vi "hardware_optpump.vi"(8 "error in":errorcluster, 10 "Pump?":bool) -> (0 "error out":errorcluster)   [LabVIEW 2012]
uses:
  <vilib>/DAQmx/write.llb/DAQmx Write (Digital Wfm 1Chan NSamp).vi
  <vilib>/Waveform/DWDTOps.llb/Digital Pattern Generator (Single Value).vi
  <vilib>/Waveform/DWDTOps.llb/DWDT Append Digital Samples.vi
  <vilib>/Waveform/DWDTOps.llb/DWDT Digital Size.vi
  <vilib>/DAQmx/create/channels.llb/DAQmx Create Channel (DO-Digital Output).vi
  <vilib>/DAQmx/configure/timing.llb/DAQmx Timing (Sample Clock).vi
  <vilib>/Waveform/DWDTOps.llb/DWDT Uncompress Digital.vi
  <vilib>/DAQmx/miscellaneous.llb/DAQmx Fill In Error Info.vi
  <resource>/objmgr/daqmx.rc
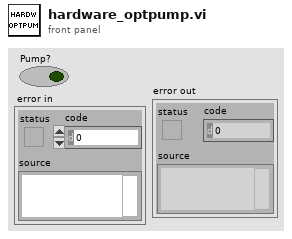
[diagram p1: front panel]
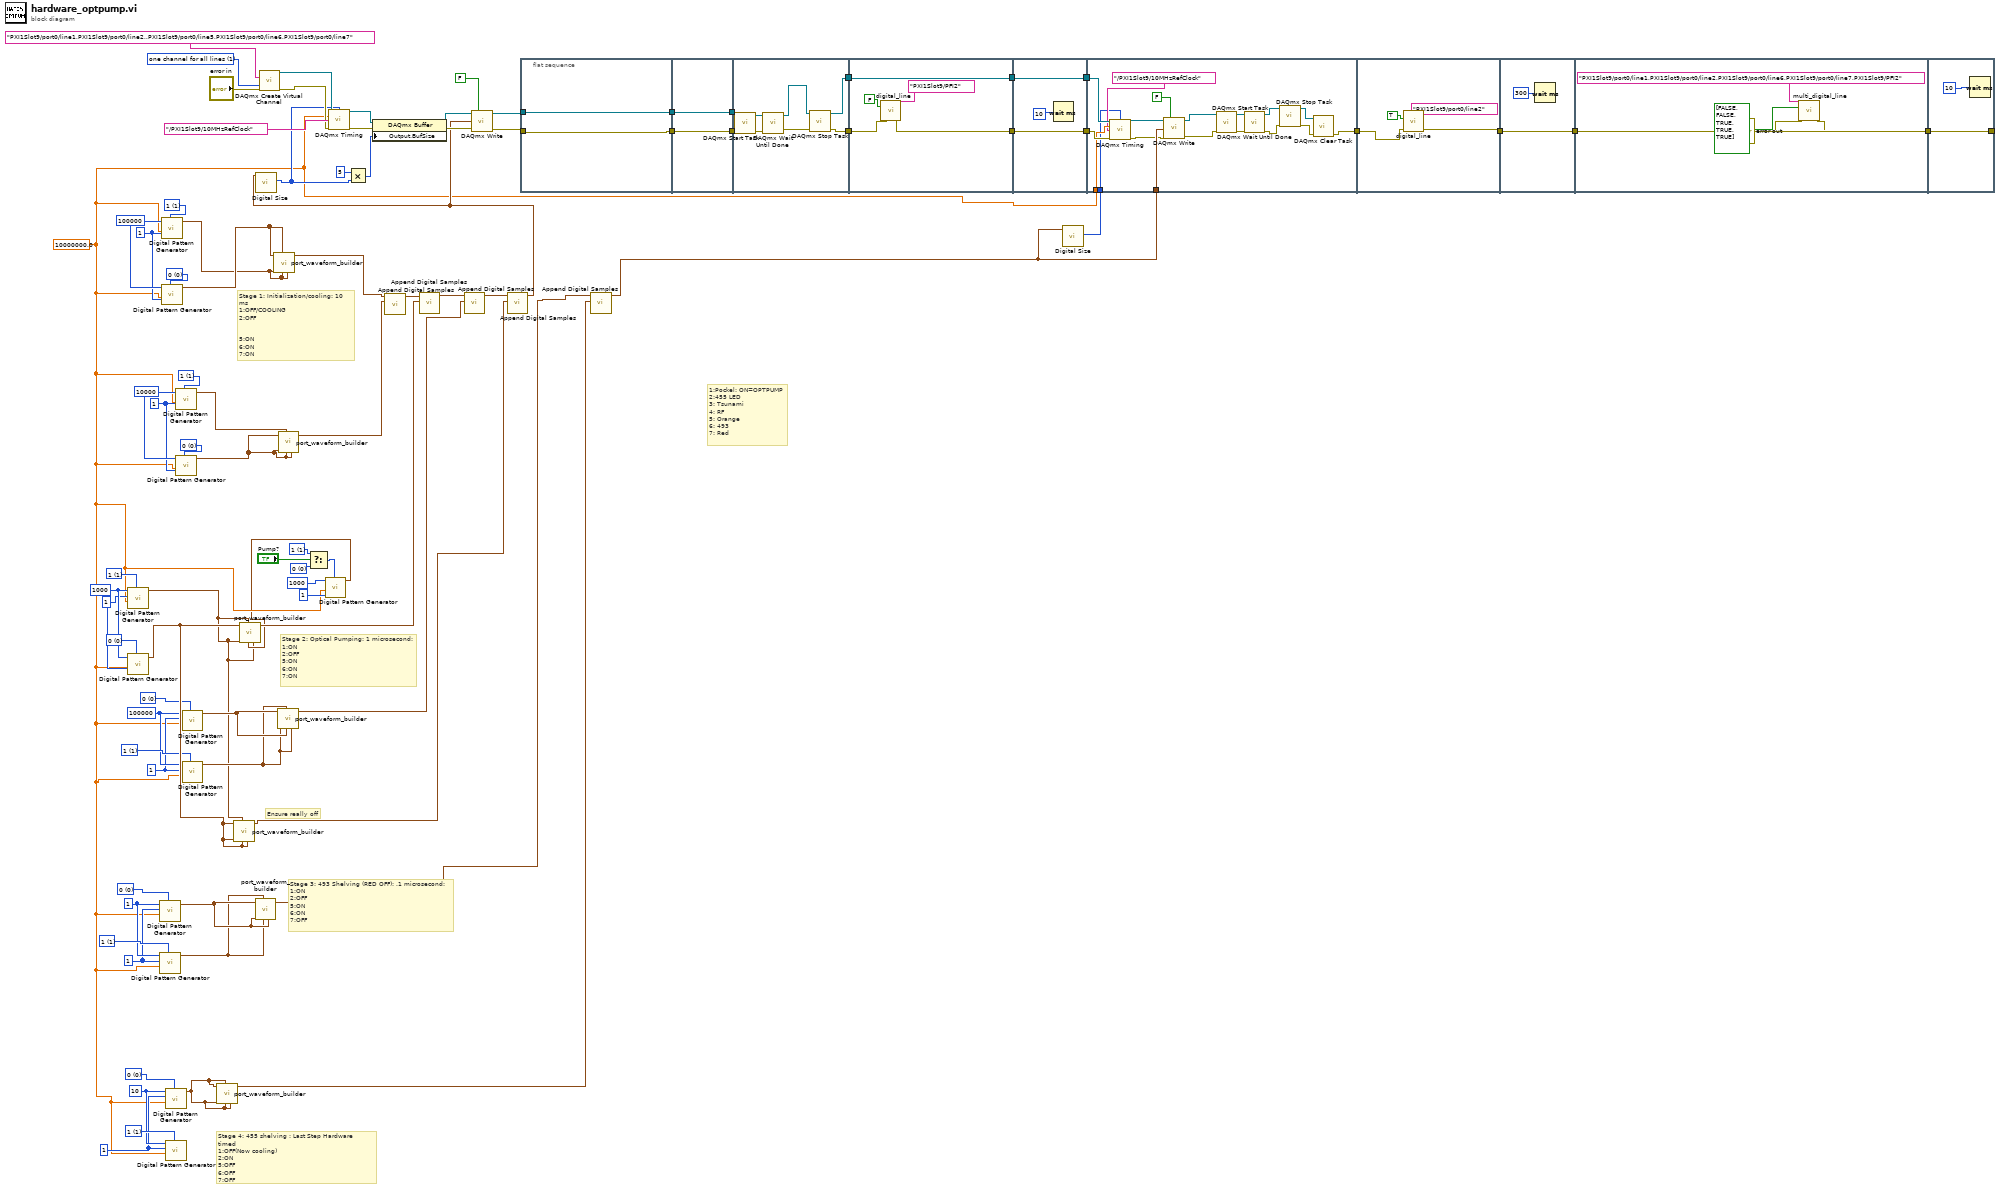
[diagram p0: block diagram]
diagram:
  w30 = u8 0 items=["0", "1", "Z", "L", "H", "X", "T", "V"] ("value")
  w28 = u32 1 ("number of signals")
  w29 = u32 100000 ("number of samples")
  w31 = u8 1 items=["0", "1", "Z", "L", "H", "X", "T", "V"] ("value")
  w44 = u8 0 items=["0", "1", "Z", "L", "H", "X", "T", "V"] ("value")
  w42 = u32 1 ("number of signals")
  w43 = u32 10000 ("number of samples")
  w45 = u8 1 items=["0", "1", "Z", "L", "H", "X", "T", "V"] ("value")
  w51 = u8 1 items=["0", "1", "Z", "L", "H", "X", "T", "V"] ("value")
  w50 = u8 0 items=["0", "1", "Z", "L", "H", "X", "T", "V"] ("value")
  w62 = u8 0 items=["0", "1", "Z", "L", "H", "X", "T", "V"] ("value")
  w60 = u32 1 ("number of signals")
  w61 = u32 10 ("number of samples")
  w63 = u8 1 items=["0", "1", "Z", "L", "H", "X", "T", "V"] ("value")
  w66 = u8 0 items=["0", "1", "Z", "L", "H", "X", "T", "V"] ("value")
  w64 = u32 1 ("number of signals")
  w65 = u32 1 ("number of samples")
  w67 = u8 1 items=["0", "1", "Z", "L", "H", "X", "T", "V"] ("value")
  w72 = u8 0 items=["0", "1", "Z", "L", "H", "X", "T", "V"] ("value")
  w68 = u32 1 ("number of signals")
  w69 = u32 1000 ("number of samples")
  w73 = u8 1 items=["0", "1", "Z", "L", "H", "X", "T", "V"] ("value")
  w74 = u8 0 items=["0", "1", "Z", "L", "H", "X", "T", "V"] ("value")
  w70 = u32 1 ("number of signals")
  w71 = u32 100000 ("number of samples")
  w75 = u8 1 items=["0", "1", "Z", "L", "H", "X", "T", "V"] ("value")
  w80 = 1 items=["one channel for each line", "one channel for all lines"] ("line grouping")
  w7 = 10000000.0 ("rate")
  # "Ensure really off"
  # "Stage 4: 455 shelving : Last Step Hardware timed\n1:OFF(Now cooling)\n2:ON\n5:OFF\n6:OFF\n7:OFF"
  # "Stage 3: 493 Shelving (RED OFF): .1 microsecond: \n1:ON\n2:OFF\n5:ON\n6:ON\n7:OFF"
  # "Stage 2: Optical Pumping: 1 microsecond: \n1:ON\n2:OFF\n5:ON\n6:ON\n7:ON"
  # "Stage 1: Initialization/cooling: 10 ms\n1:OFF/COOLING\n2:OFF\n\n\n5:ON\n6:ON\n7:ON"
  # "1:Pockel: ON=OPTPUMP\n2:455 LED\n3: Tsunami\n4: RF\n5: Orange\n6: 493\n7: Red"
  n1 = call-poly <vilib>:"Digital Pattern Generator.vi"("value"=w73, "sample rate"=w7, "number of signals"=w68, "number of samples"=w69) -> ("digital waveform"=w2:digitalwaveform)  [unwired: 6 in, 1 out]
  n2 = call-poly <vilib>:"Digital Pattern Generator.vi"("value"=w72, "sample rate"=w7, "number of signals"=w68, "number of samples"=w69) -> ("digital waveform"=w36:digitalwaveform)  [unwired: 6 in, 1 out]
  n3 = call-poly <vilib>:"Digital Pattern Generator.vi"("value"=w66, "sample rate"=w7, "number of signals"=w64, "number of samples"=w65) -> ("digital waveform"=w4:digitalwaveform)  [unwired: 6 in, 1 out]
  n4 = call-poly <vilib>:"Digital Pattern Generator.vi"("value"=w67, "sample rate"=w7, "number of signals"=w64, "number of samples"=w65) -> ("digital waveform"=w1:digitalwaveform)  [unwired: 6 in, 1 out]
  n5 = call-poly <vilib>:"Digital Pattern Generator.vi"("value"=w75, "sample rate"=w7, "number of signals"=w70, "number of samples"=w71) -> ("digital waveform"=w53:digitalwaveform)  [unwired: 6 in, 1 out]
  n6 = call-poly <vilib>:"Digital Pattern Generator.vi"("value"=w74, "sample rate"=w7, "number of signals"=w70, "number of samples"=w71) -> ("digital waveform"=w54:digitalwaveform)  [unwired: 6 in, 1 out]
  n7 = call-poly <vilib>:"Digital Pattern Generator.vi"("value"=w62, "sample rate"=w7, "number of signals"=w60, "number of samples"=w61) -> ("digital waveform"=w32:digitalwaveform)  [unwired: 6 in, 1 out]
  n8 = call-poly <vilib>:"Digital Pattern Generator.vi"("value"=w63, "sample rate"=w7, "number of signals"=w60, "number of samples"=w61) -> ()  [unwired: 6 in, 2 out]
  n9 = call-poly <vilib>:"Digital Pattern Generator.vi"("value"=w45, "sample rate"=w7, "number of signals"=w42, "number of samples"=w43) -> ("digital waveform"=w41:digitalwaveform)  [unwired: 6 in, 1 out]
  n10 = call-poly <vilib>:"Digital Pattern Generator.vi"("value"=w44, "sample rate"=w7, "number of signals"=w42, "number of samples"=w43) -> ("digital waveform"=w40:digitalwaveform)  [unwired: 6 in, 1 out]
  n11 = call-poly <vilib>:"Digital Pattern Generator.vi"("value"=w30, "sample rate"=w7, "number of signals"=w28, "number of samples"=w29) -> ("digital waveform"=w24:digitalwaveform)  [unwired: 6 in, 1 out]
  n12 = call-poly <vilib>:"Digital Pattern Generator.vi"("value"=w31, "sample rate"=w7, "number of signals"=w28, "number of samples"=w29) -> ("digital waveform"=w23:digitalwaveform)  [unwired: 6 in, 1 out]
  n13 = call "port_waveform_builder.vi"("Line 7"=w32, "Line 6"=w32, "Line 1"=w32, "Line 5"=w32, "Line 2"=w32) -> ("digital waveform out"=w58:digitalwaveform)  [unwired: 6 in]
  n14 = call "port_waveform_builder.vi"("Line 7"=w36, "Line 6"=w36, "Line 1"=w2, "Line 5"=w36, "Line 2"=w36) -> ("digital waveform out"=w35:digitalwaveform)  [unwired: 6 in]
  n15 = call "port_waveform_builder.vi"("Line 7"=w4, "Line 6"=w1, "Line 1"=w1, "Line 5"=w4, "Line 2"=w4) -> ("digital waveform out"=w15:digitalwaveform)  [unwired: 6 in]
  n16 = call-poly <vilib>:"DAQmx Create Virtual Channel.vi"("lines"=tag "PXI1Slot9/port0/line1,PXI1Slot9/port0/line2,,PXI1Slot9/port0/line5,PXI1Slot9/port0/line6,PXI1Slot9/port0/line7", "line grouping"=w80, "error in"="error in") -> ("task out"=w81:refnum<k21>, "error out"=w78:errorcluster)  [unwired: 11 in]
  n17 = call "port_waveform_builder.vi"("Line 7"=w53, "Line 6"=w53, "Line 1"=w54, "Line 5"=w53, "Line 2"=w54) -> ("digital waveform out"=w39:digitalwaveform)  [unwired: 6 in]
  n18 = call "port_waveform_builder.vi"("Line 7"=w23, "Line 6"=w24, "Line 1"=w23, "Line 5"=w23, "Line 2"=w24) -> ("digital waveform out"=w25:digitalwaveform)  [unwired: 6 in]
  n19 = call "port_waveform_builder.vi"("Line 7"=w40, "Line 6"=w40, "Line 1"=w41, "Line 5"=w40, "Line 2"=w40) -> ("digital waveform out"=w38:digitalwaveform)  [unwired: 6 in]
  n20 = Select(t=w51, s="Pump?", f=w50) -> (s? t:f=w47:u8)
  n21 = call-poly <vilib>:"Digital Pattern Generator.vi"("value"=w47, "sample rate"=w7, "number of signals"=u32 1, "number of samples"=u32 1000) -> ("digital waveform"=w3:digitalwaveform)  [unwired: 6 in, 1 out]
  n22 = call "port_waveform_builder.vi"("Line 7"=w2, "Line 6"=w3, "Line 1"=w2, "Line 5"=w2, "Line 2"=w36) -> ("digital waveform out"=w59:digitalwaveform)  [unwired: 6 in]
  n23 = call-poly <vilib>:"Append Digital Samples.vi"("digital waveform B"=w38, "digital waveform A"=w39) -> ("digital waveform out"=w37:digitalwaveform)  [unwired: 8 in, 1 out]
  n24 = call-poly <vilib>:"Append Digital Samples.vi"("digital waveform B"=w59, "digital waveform A"=w37) -> ("digital waveform out"=w27:digitalwaveform)  [unwired: 8 in, 1 out]
  n25 = call-poly <vilib>:"Append Digital Samples.vi"("digital waveform B"=w25, "digital waveform A"=w27) -> ("digital waveform out"=w26:digitalwaveform)  [unwired: 8 in, 1 out]
  n26 = call-poly <vilib>:"Append Digital Samples.vi"("digital waveform B"=w35, "digital waveform A"=w26) -> ("digital waveform out"=w14:digitalwaveform)  [unwired: 8 in, 1 out]
  n27 = call-poly <vilib>:"Digital Size.vi"("digital waveform in"=w14) -> ("number of samples"=w8:i32)  [unwired: 7 in, 3 out]
  n28 = call-poly <vilib>:"DAQmx Timing.vi"("task/channels in"=w81, "samples per channel"=w8, "rate"=w7, "source"=tag "/PXI1Slot9/10MHzRefClock", "error in"=w78) -> ("task out"=w86:refnum<k21>, "error out"=w85:errorcluster)  [unwired: 9 in]
  n29 = Multiply(x=5, y=w8) -> (x*y=w17:i32)
  n30 = property class="DAQmx Buffer"(reference=w86, error in=w85, "Output.BufSize"=w17) -> (reference out=w83:refnum<k21>, error out=w77:errorcluster)
  n31 = call-poly <vilib>:"DAQmx Write.vi"("task/channels in"=w83, "auto start"=FALSE, "data"=w14, "error in"=w77) -> ("task out"=w82:refnum<k21>, "error out"=w76:errorcluster)  [unwired: 9 in, 1 out]
  n32 = flat-sequence {
    tunnel: w76 -> [w88]
    tunnel: w82 -> [w89]
    tunnel: [w89] -> w21
    tunnel: [w88] -> w18
    tunnel: w21 -> [w91]
    tunnel: [w91] -> w20
    tunnel: [w90] -> w19
    tunnel: w18 -> [w90]
    tunnel: w20 -> [w99]
    tunnel: w19 -> [w98]
    tunnel: [w95] -> w10
    tunnel: [w94] -> w9
    tunnel: [w104] -> w34
    tunnel: [w100] -> w11
    tunnel: w10 -> [w100]
    tunnel: w9 -> [w103]
    tunnel: w34 -> [w107]
    tunnel: [w107] -> w16
    tunnel: [w105] -> w12
    tunnel: w11 -> [w105]
    tunnel: w16 -> [w114]
    tunnel: [w115] -> w13
    tunnel: w12 -> [w111]
    tunnel: w6 -> [w125]
    tunnel: w7 -> [w110]
    tunnel: w5 -> [w108]
    tunnel: [w126] -> w33
    tunnel: w13 -> [w127]
    tunnel: w33 -> [w131]
    tunnel: [w131] -> w52
    tunnel: w52 -> [w135]
    tunnel: [w134] -> w22
    tunnel: [w137] -> w56
    tunnel: w22 -> [w137]
    frame #0 {
    }
    frame #1 {
    }
    frame #2 {
      n33 = call <vilib>:"DAQmx Start Task.vi"("task/channels in"=w99, "error in"=w98) -> ("task out"=w96:refnum<k21>, "error out"=w97:errorcluster)  [unwired: 12 in]
      n34 = call <vilib>:"DAQmx Wait Until Done.vi"("task/channels in"=w96, "error in"=w97) -> ("task out"=w92:refnum<k21>, "error out"=w93:errorcluster)  [unwired: 12 in]
      n35 = call <vilib>:"DAQmx Stop Task.vi"("task/channels in"=w92, "error in"=w93) -> ("task out"=w95:refnum<k21>, "error out"=w94:errorcluster)  [unwired: 12 in]
    }
    frame #3 {
      n36 = call "digital_line.vi"("error in"=w103, "Boolean"=FALSE, "lines"=tag "PXI1Slot9/PFI2") -> ("error out"=w104:errorcluster)  [unwired: 4 in]
    }
    frame #4 {
      n37 = Wait (ms)(milliseconds to wait=u32 10) -> ()  [unwired: 1 out]
    }
    frame #5 {
      n38 = call-poly <vilib>:"DAQmx Timing.vi"("task/channels in"=w111, "samples per channel"=w108, "rate"=w110, "source"=tag "/PXI1Slot9/10MHzRefClock", "error in"=w114) -> ("task out"=w112:refnum<k21>, "error out"=w113:errorcluster)  [unwired: 9 in]
      n39 = call-poly <vilib>:"DAQmx Write.vi"("task/channels in"=w112, "auto start"=FALSE, "data"=w125, "error in"=w113) -> ("task out"=w123:refnum<k21>, "error out"=w116:errorcluster)  [unwired: 9 in, 1 out]
      n40 = call <vilib>:"DAQmx Start Task.vi"("task/channels in"=w123, "error in"=w116) -> ("task out"=w122:refnum<k21>, "error out"=w117:errorcluster)  [unwired: 12 in]
      n41 = call <vilib>:"DAQmx Wait Until Done.vi"("task/channels in"=w122, "error in"=w117) -> ("task out"=w121:refnum<k21>, "error out"=w118:errorcluster)  [unwired: 12 in]
      n42 = call <vilib>:"DAQmx Stop Task.vi"("task/channels in"=w121, "error in"=w118) -> ("task out"=w120:refnum<k21>, "error out"=w119:errorcluster)  [unwired: 12 in]
      n43 = call <vilib>:"DAQmx Clear Task.vi"("task in"=w120, "error in"=w119) -> ("error out"=w115:errorcluster)  [unwired: 13 in]
    }
    frame #6 {
      n44 = call "digital_line.vi"("error in"=w127, "Boolean"=TRUE, "lines"=tag "PXI1Slot9/port0/line2") -> ("error out"=w126:errorcluster)  [unwired: 4 in]
    }
    frame #7 {
      n45 = Wait (ms)(milliseconds to wait=u32 300) -> ()  [unwired: 1 out]
    }
    frame #8 {
      n46 = call "multi_digital_line.vi"("error in"=w135, "data"=bool[] [FALSE, FALSE, TRUE, TRUE, TRUE], "lines"=tag "PXI1Slot9/port0/line1,PXI1Slot9/port0/line2,PXI1Slot9/port0/line6,PXI1Slot9/port0/line7,PXI1Slot9/PFI2") -> ("error out"=w134:errorcluster)  [unwired: 8 in]
    }
    frame #9 {
      n47 = Wait (ms)(milliseconds to wait=u32 10) -> ()  [unwired: 1 out]
    }
  }
  n48 = call-poly <vilib>:"Append Digital Samples.vi"("digital waveform B"=w58, "digital waveform A"=w15) -> ("digital waveform out"=w6:digitalwaveform)  [unwired: 8 in, 1 out]
  n49 = call-poly <vilib>:"Digital Size.vi"("digital waveform in"=w6) -> ("number of samples"=w5:i32)  [unwired: 7 in, 3 out]
  "error out" <- w56
